vi "LabviewC#101.vi"() -> ()   [LabVIEW 2017]
uses:
  C:/Users/GB/Desktop/LabviewC#dll/ClassLibrary1/ClassLibrary1/bin/Debug/ClassLibrary1.dll
  ClassLibrary1/ClassLibrary1/bin/Debug/ClassLibrary1.dll
panel:
  out "minus":dbl
  out "addup":dbl
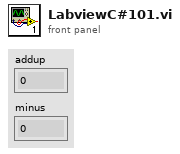
[diagram p1: front panel]
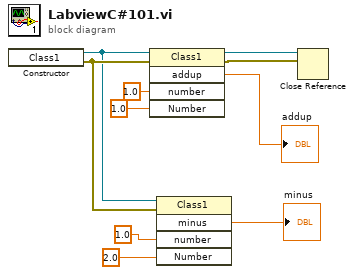
[diagram p0: block diagram]
diagram:
  n1 = constructor class="Class1"() -> (reference out=w4:refnum<k24>, error out=w5:errorcluster)  [unwired: 3 in, 1 out]
  n2 = invoke class="Class1" method="addup"(reference=w4, error in=w5, "number"=1.0, "Number"=1.0) -> (reference out=w10:refnum<k24>, error out=w9:errorcluster, "addup"=→"addup":dbl)  [unwired: 1 in, 2 out]
  n3 = invoke class="Class1" method="minus"(reference=w4, error in=w5, "number"=1.0, "Number"=2.0) -> ("minus"=→"minus":dbl)  [unwired: 1 in, 4 out]
  n4 = Close Reference(reference=w10, error in (no error)=w9) -> ()  [unwired: 1 out]
